vi "Set Initialization Data - Place Temperature.vi"(7 "Show Frontpanel":bool, 8 "error in":errorcluster, 11 "Controller in":refnum<class "Controller.lvclass">) -> (0 "error out":errorcluster, 3 "Controller out":refnum<class "Controller.lvclass">)   [LabVIEW 2024, in "Controller.lvclass"]
doc: "In this VI you can set the initialization data of a statically-linked subWorker."
uses:
  Controller.lvclass
  Place Temperature/Initialization Data.ctl
  Controller.lvclass/Controller.ctl
  Place Temperature/Place Temperature.lvclass
  C:/Program Files (x86)/National Instruments/LabVIEW 2024/vi.lib/addons/_Workers/Library/Classes/Worker/Worker.lvclass
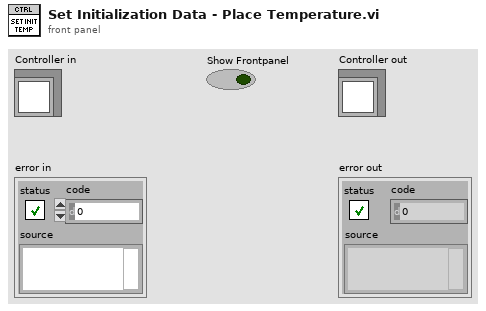
[diagram p1: front panel]
types:
  T1 = typedef "Place Temperature.lvclass/Initialization Data.ctl" = cluster{"String":string, "Show Frontpanel":bool}
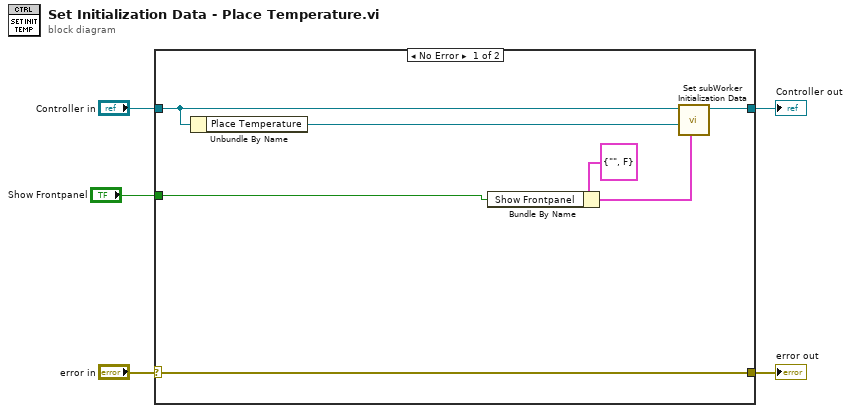
[diagram p0: block diagram]
diagram:
  n1 = case shown="No Error" "error in" {
    selector: "error in" -> [w12 w14]
    tunnel: [w12 w14] -> w4
    tunnel: [w10 w13] -> w3
    tunnel: "Controller in" -> [w9 w13]
    tunnel: "Show Frontpanel" -> [w6 _]
    frame No Error {
      n2 = Unbundle By Name(w9) -> ("Place Temperature"=w11:refnum<class "Place Temperature.lvclass">)
      n3 = Bundle By Name(cluster=T1 {"String"="", "Show Frontpanel"=FALSE} ("Initialization Data"), "Show Frontpanel"=w6) -> (w7:T1)
      n4 = call-dynamic "Set subWorker Initialization Data.vi"("Initialization Data"=w7, "subWorker"=w11, "Worker"=w9) -> ("Worker out"=w10:refnum<class "Controller.lvclass">)  [unwired: 8 in]
    }
    frame Error {
    }
  }
  "error out" <- w4
  "Controller out" <- w3
